vi "Read Max Sample Rate.vi"(8 "error in (no error)":errorcluster, 11 "Oscilloscope in":refnum<class "Oscilloscope.lvclass">) -> (0 "error out":errorcluster, 2 "Max Sample Rate":dbl, 3 "Oscilloscope out":refnum<class "Oscilloscope.lvclass">)   [LabVIEW 2019, in "Oscilloscope.lvlib" / "Oscilloscope.lvclass"]
uses:
  Oscilloscope.lvclass
  Oscilloscope.lvclass/Oscilloscope.ctl
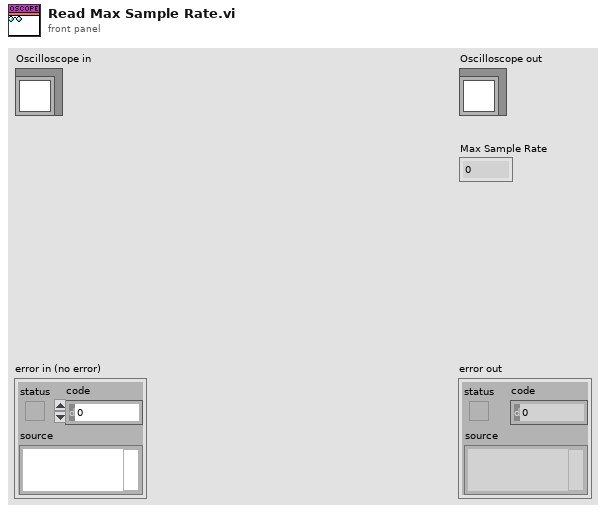
[diagram p1: front panel]
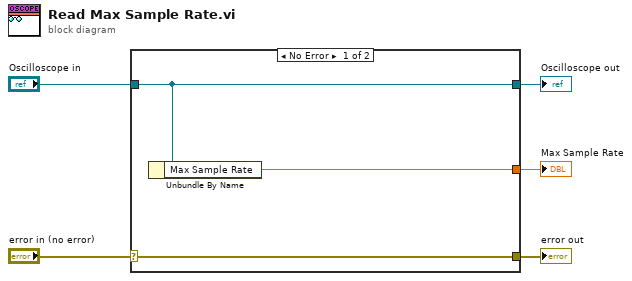
[diagram p0: block diagram]
diagram:
  n1 = case shown="No Error" "error in (no error)" {
    selector: "error in (no error)" -> [w8 w9]
    tunnel: [w8 w9] -> w4
    tunnel: [w7 w10] -> w2
    tunnel: "Oscilloscope in" -> [w7 w10]
    tunnel: [w6 _] -> w1
    frame No Error {
      n2 = Unbundle By Name(w7) -> ("Max Sample Rate"=w6:dbl)
    }
    frame Error {
    }
  }
  "error out" <- w4
  "Oscilloscope out" <- w2
  "Max Sample Rate" <- w1
